vi "Display Image.vi"(11 "Image 2":T1(plugin-control)) -> ()   [LabVIEW 2012]
uses:
  Global variables.vi
panel:
  out "Image":T1(plugin-control)
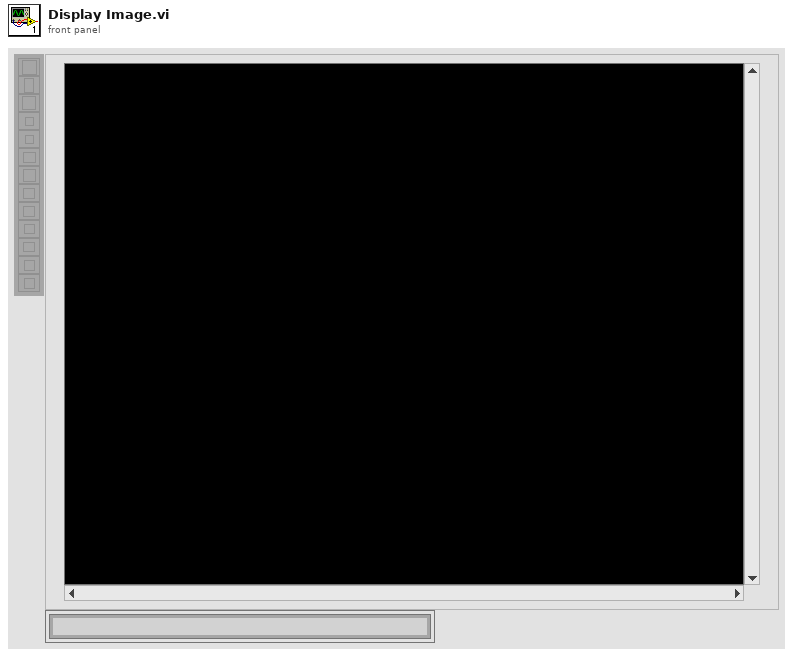
[diagram p1: front panel]
types:
  T1 = typedef "IMAQ Image.ctl" = refnum<image>
  T2 = cluster{"Global Rectangle":i32[], "Contours":cluster{"Contour Type":u32, "ROI Type":u32, "Points":i32[]}[]}
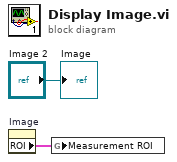
[diagram p0: block diagram]
diagram:
  n1 = property on="Image" class="ImageControl"() -> ("ROI"=w1:T2)  [unwired: 2 in, 2 out]
  n2 = global write "Global variables.vi" "Measurement ROI"(w1) -> ()
  "Image" <- "Image 2"
